vi "DHE_DRV_set_mapsize.vi"(7 "size_MB":i32, 11 "error in (no error)":errorcluster) -> (8 "return value":i32, 15 "error out":errorcluster)   [LabVIEW 2016]
doc: "This VI closes the I/O interface with the instrument."
uses:
  c/lib/libarcDHE.so
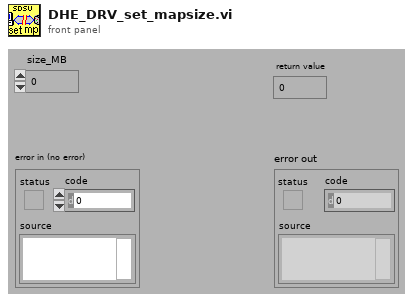
[diagram p1: front panel]
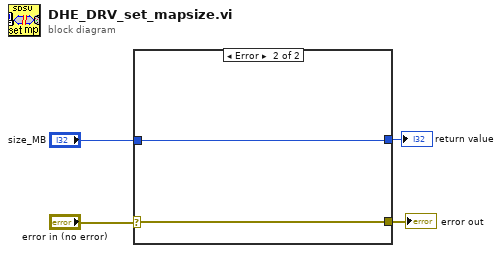
[diagram p0: block diagram]
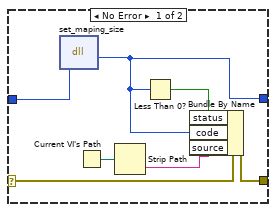
[diagram p2: hidden frame]
diagram:
  n1 = case shown="Error" "error in (no error)" {
    selector: "error in (no error)" -> [w5 w12]
    tunnel: [w10 w13] -> w4
    tunnel: [w7 w12] -> w3
    tunnel: "size_MB" -> [w6 w13]
    frame No Error {
      n2 = dll-call lib="home/simager/panview/PAN/Modules/SDSU/private/c/lib/libarcDHE.so" fn="set_maping_size"("size_MB"=w6) -> ("return type"=w10:i32)  [unwired: 4 in, 2 out]
      n3 = Current VI's Path() -> (path=w9:path)
      n4 = Strip Path(path=w9) -> (name=w8:string)  [unwired: 1 out]
      n5 = Less Than 0?(x=w10) -> (x < 0?=w11:bool)
      n6 = Bundle By Name(cluster=w5, "status"=w11, "code"=w10, "source"=w8) -> (w7:errorcluster)
    }
    frame Error {
    }
  }
  "error out" <- w3
  "return value" <- w4
